vi "Cannon Set.vi"(1 "Cannon Info In":T2) -> (0 "Cannon Info Out":T2)   [LabVIEW 2013]
uses:
  <vilib>/Rock Robotics/WPI/Relay/WPI_RelayValue.ctl
  Intake/Intake Global.vi
  <vilib>/Rock Robotics/WPI/Solenoid/WPI_SolenoidSetEnum.vi
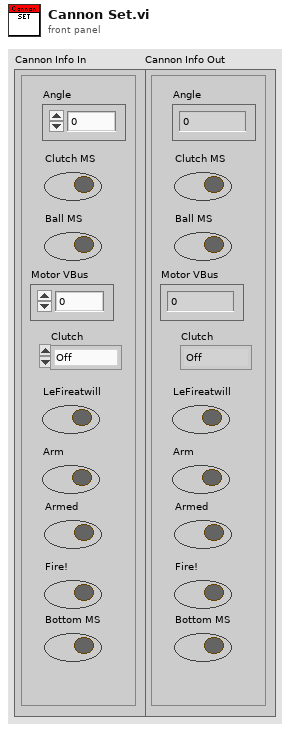
[diagram p1: front panel]
types:
  T1 = typedef "WPI_RelayValue.ctl" = enum16{"Off", "On", "Forward", "Reverse"}
  T2 = cluster{"Angle":dbl, "Clutch MS":bool, "Ball MS":bool, "Clutch ":T1, "LeFireatwill":bool, "Arm":bool, "Armed":bool, "Fire!":bool, "Bottom MS":bool, "Motor VBus":dbl}
  T3 = typedef "WPI_SolenoidValue.ctl" = enum16{"Off", "On", "Forward", "Reverse"}
  T4 = cluster{"Arm State":bool, "Gripper Out":bool, "Gripper Execution":T1, "Arm Execution":T3, "Gripper In":bool}
  T5 = typedef "WPI_MotorControlDeviceRef.ctl" = cluster{"DeviceStatus":errorcluster, "Type":enum16{"PWM", "CAN"}, "PWM":cluster{"Digital Module":T6, "PWM Channel":T7, "DeadBand":T8}, "CAN":cluster{"Device Number":u8, "Control Mode":T9, "Semaphore":T10, "Max Vout":dbl}, "Invert":bool, "TransformRef":T11, "InvTransformRef":T11}
  T6 = typedef "FPGA_TypedefDigitalModule.ctl" = enum16{"Digital Module 1", "Digital Module 2"}
  T7 = typedef "FPGA_DIOPWMChannel.ctl" = enum8{"PWM 1", "PWM 2", "PWM 3", "PWM 4", "PWM 5", "PWM 6", "PWM 7", "PWM 8", "PWM 9", "PWM 10", "Invalid"}
  T8 = typedef "WPI_PWMDeadband.ctl" = cluster{"Name":string, "maxPositivePwm":i32, "minPositivePwm":i32, "centerPwm":i32, "maxNegativePwm":i32, "minNegativePwm":i32, "angularRange":u16}
  T9 = typedef "WPI_CANJaguar_ControlMode.ctl" = enum8{"Percent VBus", "Current", "Speed", "Position", "Voltage"}
  T10 = typedef "Semaphore RefNum" = refnum<k1>
  T11 = typedef "WPI_PWMTransform_ConPane.ctl" = refnum<vi>
  T12 = typedef "WPI_SolenoidDevRef.ctl" = cluster{"DevStatus":errorcluster, "Solenoid Module":T13, "Forward Solenoid Channel":T14, "Reverse Solenoid Channel":T14}
  T13 = typedef "FPGA_TypedefSolenoidModule.ctl" = enum16{"Solenoid Module 1", "Solenoid Module 2"}
  T14 = typedef "WPI_SolenoidChannel.ctl" = enum8{"Solenoid 1", "Solenoid 2", "Solenoid 3", "Solenoid 4", "Solenoid 5", "Solenoid 6", "Solenoid 7", "Solenoid 8", "Invalid"}
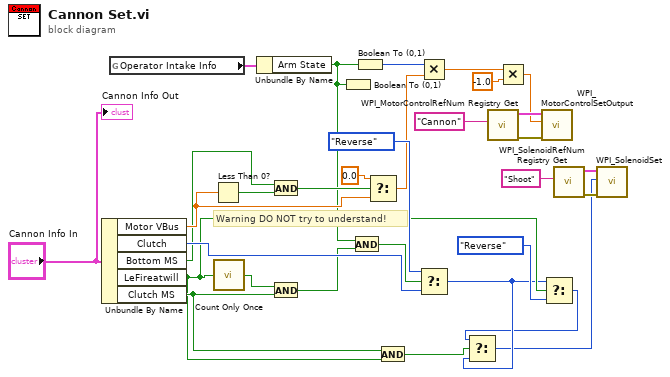
[diagram p0: block diagram]
diagram:
  # "Warning DO NOT try to understand!"
  n1 = Unbundle By Name("Cannon Info In") -> ("Motor VBus"=w17:dbl, "Clutch"=w23:T1, "Bottom MS"=w1:bool, "LeFireatwill"=w6:bool, "Clutch MS"=w7:bool)
  n2 = global read "Intake Global.vi" "Operator Intake Info"() -> (w25:T4)
  n3 = Less Than 0?(x=w17) -> (x < 0?=w20:bool)
  n4 = call "Count Only Once.vi"("InValue"=w6) -> ("Result"=w16:bool)
  n5 = Unbundle By Name(w25) -> ("Arm State"=w14:bool)
  n6 = And(x=w1, y=w20) -> (x .and. y?=w19:bool)
  n7 = And(x=w16, y=w7) -> (x .and. y?=w22:bool)
  n8 = Boolean To (0,1)(Boolean=w14) -> ()  [unwired: 1 out]
  n9 = And(x=w14, y=w22) -> (x .and. y?=w21:bool)
  n10 = Boolean To (0,1)(Boolean=w14) -> (0, 1=w15:i16)
  n11 = Select(t=0.0 ("f"), s=w19, f=w17) -> (s? t:f=w13:dbl)
  n12 = And(x=w7, y=w6) -> (x .and. y?=w5:bool)
  n13 = Multiply(x=w15, y=w13) -> (x*y=w11:dbl)
  n14 = Select(t=WPI_RelayValue."Reverse" ("y"), s=w21, f=w23) -> (s? t:f=w4:T1)
  n15 = call <vilib>:"WPI_MotorControlRefNum Registry Get.vi"("refnum name"="Cannon") -> ("error out"=w28:errorcluster, "MotorControlDevRef"=w29:T5)  [unwired: 9 in]
  n16 = Multiply(x=w11, y=-1.0) -> (x*y=w9:dbl)
  n17 = call <vilib>:"WPI_MotorControlSetOutput.vi"("error in (no error)"=w28, "Output"=w9, "MotorControlDevRef"=w29) -> ()  [unwired: 6 in, 3 out]
  n18 = Select(t=w4, s=w6, f=WPI_RelayValue."Reverse" ("y")) -> (s? t:f=w3:T1)
  n19 = Select(t=w3, s=w5, f=w4) -> (s? t:f=w2:T1)
  n20 = call <vilib>:"WPI_SolenoidRefNum Registry Get.vi"("refnum name"="Shoot") -> ("error out"=w30:errorcluster, "SolenoidDevRef"=w31:T12)  [unwired: 9 in]
  n21 = call-poly <vilib>:"WPI_SolenoidSet.vi"("error in (no error)"=w30, "Value"=w2, "SolenoidDevRef"=w31) -> ()  [unwired: 7 in, 2 out]
  "Cannon Info Out" <- "Cannon Info In"
